vi "Analysis.Data Dump, Result Header to to 1D Str_V3.vi"(10 "Result Summary":T1, 11 "Header Names":string[](array[string])=["FP", "LP", "SN", "Start Time", "Location", "Nest", "Sequence", "Test Mode", "Operator", "Comment", "Result", "Result Code", "Result Desc", "Duration(s)"]) -> (3 "Data List out":string[](array[string]))   [LabVIEW 2024]
uses:
  Analysis.Result Summary_V2.ctl
  Analysis.Data Value Items Action.ctl
  Time/Time.Format Selector.ctl
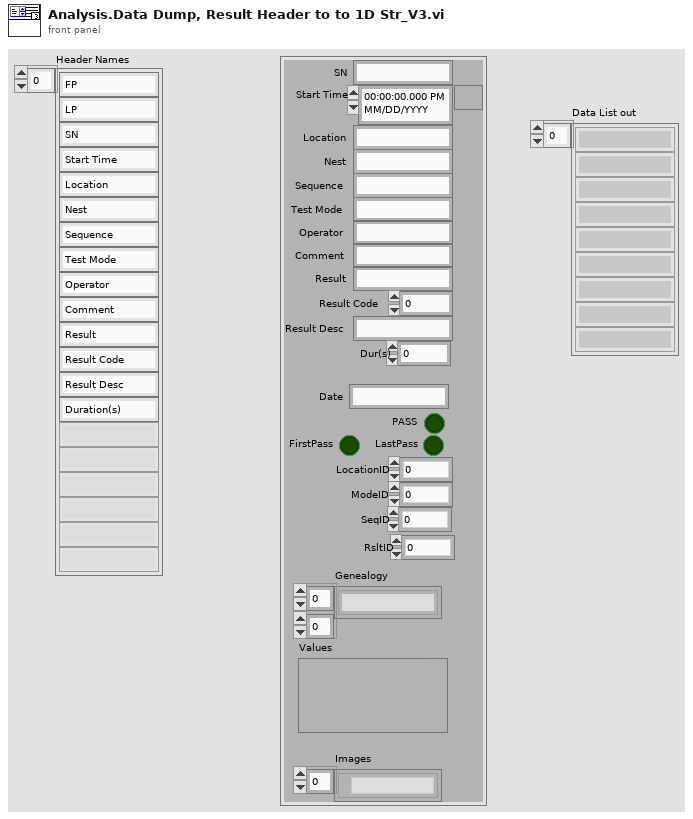
[diagram p1: front panel]
types:
  T1 = typedef "Analysis.Result Summary_V2.ctl" = cluster{"SN":string, "Start Time":timestamp, "Location":string, "Nest":string, "Sequence":string, "Operator":string, "Test Mode":string, "Comment":string, "Result":string, "Result Code":i32, "Result Desc":string, "Date":string, "Dur(s)":dbl, "PASS":bool, "FirstPass":bool, "LastPass":bool, "LocationID":i32, "ModeID":i32, "SeqID":i32, "RsltID":i32, "Genealogy":string[][], "Values":variant, "Images":path[]}
  T2 = typedef "Analysis.Data Value Items Action.ctl" = enum16{"Init", "Add Value", "Get MeasVals", "Get Lists", "Get RsltVals", "Dump All", "Dump Vals to File", "Get Rslt Meas Val", "Dump Lists to File", "Load Values from File", "Load Lists From File", "Get MeasVals Num Only", "TrimDataTable"}
  T3 = typedef "Time.Format Selector.ctl" = enum16{"yyyy/mm/dd HH:MM:S.sss", "yyyy/mm/dd HH:MM:SS", "yyyy-MM-ddTHH:mm:ss[.mmm]", "YYYYMMDD_HHMMSS"}
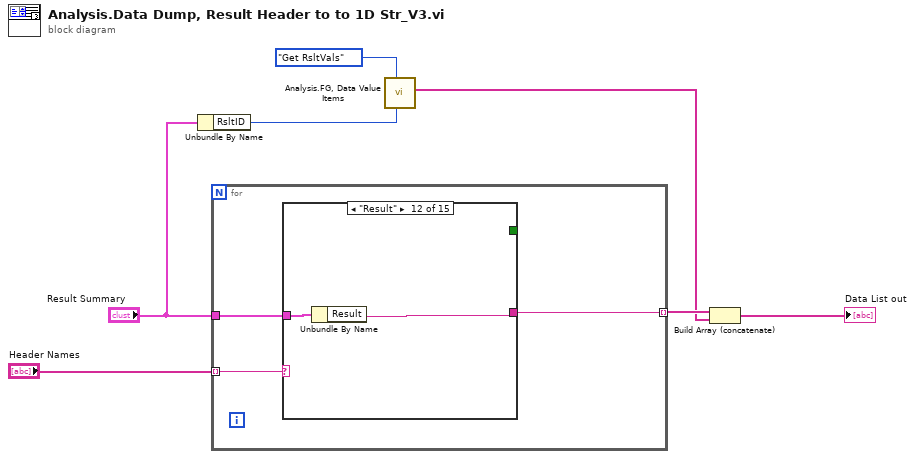
[diagram p0: block diagram]
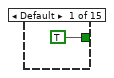
[diagram p2: hidden frame]
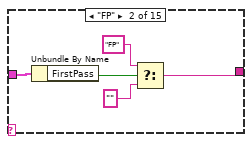
[diagram p3: hidden frame]
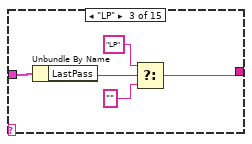
[diagram p4: hidden frame]
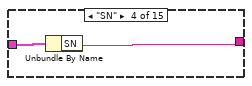
[diagram p5: hidden frame]
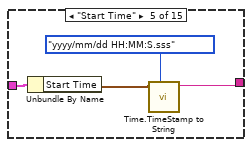
[diagram p6: hidden frame]
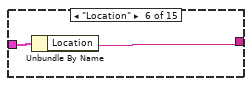
[diagram p7: hidden frame]
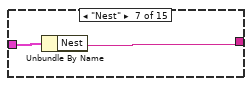
[diagram p8: hidden frame]
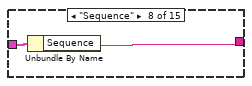
[diagram p9: hidden frame]
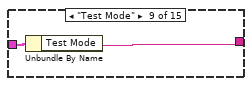
[diagram p10: hidden frame]
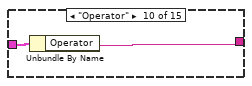
[diagram p11: hidden frame]
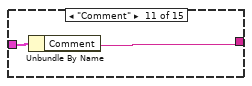
[diagram p12: hidden frame]
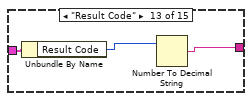
[diagram p13: hidden frame]
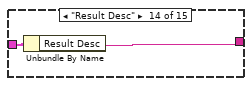
[diagram p14: hidden frame]
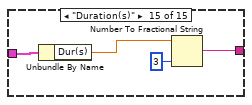
[diagram p15: hidden frame]
diagram:
  n1 = Unbundle By Name("Result Summary") -> ("RsltID"=w5:i32)
  n2 = for {
    tunnel: "Result Summary" -> [w10]
    tunnel: "Header Names" -> [w9] mode=indexing
    tunnel: [w8] -> w3 mode=indexing
    n3 = case shown="\"Result\"" w9 {
      tunnel: [_ w14 w19 w22 w25 w28 w30 w32 w34 w36 w38 w40 w42 w45 w47] -> w8
      tunnel: w10 -> [_ w16 w21 w23 w27 w29 w31 w33 w35 w37 w39 w41 w44 w46 w50]
      tunnel: [TRUE _ _ _ _ _ _ _ _ _ _ _ _ _ _] -> _
      frame Default {
      }
      frame "FP" {
        n4 = Unbundle By Name(w16) -> ("FirstPass"=w15:bool)
        n5 = Select(t="FP", s=w15, f="") -> (s? t:f=w14:string)
      }
      frame "LP" {
        n6 = Unbundle By Name(w21) -> ("LastPass"=w20:bool)
        n7 = Select(t="LP", s=w20, f="") -> (s? t:f=w19:string)
      }
      frame "SN" {
        n8 = Unbundle By Name(w23) -> ("SN"=w22:string)
      }
      frame "Start Time" {
        n9 = Unbundle By Name(w27) -> ("Start Time"=w26:timestamp)
        n10 = call "Time.TimeStamp to String.vi"("TimeFormat"=Time.Format_Selector."yyyy/mm/dd HH:MM:S.sss", "Time Stamp in"=w26) -> ("Time String Out"=w25:string)  [unwired: 9 in]
      }
      frame "Location" {
        n11 = Unbundle By Name(w29) -> ("Location"=w28:string)
      }
      frame "Nest" {
        n12 = Unbundle By Name(w31) -> ("Nest"=w30:string)
      }
      frame "Sequence" {
        n13 = Unbundle By Name(w33) -> ("Sequence"=w32:string)
      }
      frame "Test Mode" {
        n14 = Unbundle By Name(w35) -> ("Test Mode"=w34:string)
      }
      frame "Operator" {
        n15 = Unbundle By Name(w37) -> ("Operator"=w36:string)
      }
      frame "Comment" {
        n16 = Unbundle By Name(w39) -> ("Comment"=w38:string)
      }
      frame "Result" {
        n17 = Unbundle By Name(w41) -> ("Result"=w40:string)
      }
      frame "Result Code" {
        n18 = Unbundle By Name(w44) -> ("Result Code"=w43:i32)
        n19 = Number To Decimal String(number=w43) -> (decimal integer string=w42:string)  [unwired: 1 in]
      }
      frame "Result Desc" {
        n20 = Unbundle By Name(w46) -> ("Result Desc"=w45:string)
      }
      frame "Duration(s)" {
        n21 = Unbundle By Name(w50) -> ("Dur(s)"=w49:dbl)
        n22 = Number To Fractional String(number=w49, precision (6)=i16 3) -> (F-format string=w47:string)  [unwired: 2 in]
      }
    }
  }
  n23 = call "Analysis.FG, Data Value Items.vi"("ResultID"=w5, "Action"=Analysis.Data_Value_Items_Action."Get RsltVals") -> ("Name/1DVals Out"=w2:string[])  [unwired: 5 in, 4 out]
  n24 = Build Array (concatenate)(w3, w2) -> (→"Data List out":string[])
